vi "sonar_movement.vi"() -> ()   [LabVIEW 2014]
uses:
  <vilib>/NXT/Subs/MotorOutput.ctl
panel:
  out "P2 (dB) 2":i16
  out "P1 (dB)":i16
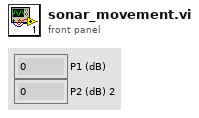
[diagram p1: front panel]
types:
  T1 = typedef "MotorOutput.ctl" = u8
  T2 = typedef "LVHSConnector.ctl" = refnum<class "BrickReference.lvclass">
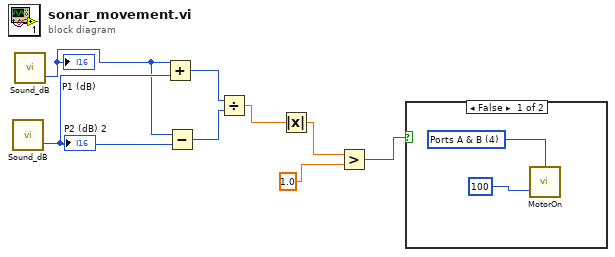
[diagram p0: block diagram]
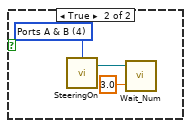
[diagram p2: hidden frame]
diagram:
  n1 = call <vilib>:"Sound_dB.vi"() -> ("Sound (dB)"=w8:i16)  [unwired: 3 in, 1 out]
  "P2 (dB) 2" <- w8
  n2 = call <vilib>:"Sound_dB.vi"() -> ("Sound (dB)"=w7:i16)  [unwired: 3 in, 1 out]
  "P1 (dB)" <- w7
  n3 = Add(x=w7, y=w8) -> (x+y=w6:i16)
  n4 = Subtract(x=w7, y=w8) -> (x-y=w5:i16)
  n5 = Divide(x=w6, y=w5) -> (x/y=w4:dbl)
  n6 = Absolute Value(x=w4) -> (abs(x)=w1:dbl)
  n7 = Greater?(x=w1, y=1.0) -> (0:w3:bool)
  n8 = case shown="False" w3 {
    frame False {
      w10 = T1 4 items=["Port A"=0, "Port B"=1, "Port C"=2, "Ports A & B"=4, "Ports A & C"=5, "Ports B & C"=6, "All Ports"=3] ("Output Port (All Ports)")
      n9 = call <vilib>:"MotorOn.vi"("Power (75)"=100, "Output Port (All Ports)"=w10) -> ()  [unwired: 2 in, 1 out]
    }
    frame True {
      w13 = T1 4 items=["Port A"=0, "Port B"=1, "Port C"=2, "Ports A & B"=4, "Ports A & C"=5, "Ports B & C"=6, "All Ports"=3] ("Output Ports (A & B)")
      n10 = call <vilib>:"SteeringOn.vi"("Output Ports (A & B)"=w13) -> ("NXT/EV3"=w12:T2)  [unwired: 3 in]
      n11 = call <vilib>:"Wait_Num.vi"("Time (1 sec)"=sgl 3.0, "NXT/EV3"=w12) -> ()  [unwired: 2 in, 1 out]
    }
  }
